vi "5492_InitialYaw.vi"() -> ()   [LabVIEW 2016]
panel:
  in  "INITIAL\n YAW":dbl
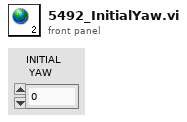
[diagram p1: front panel]
diagram:
